vi "Receiver.vi"() -> ()   [LabVIEW 2019]
uses:
  <vilib>/httpClient/LabVIEWHTTPClient.lvlib
  <vilib>/smtpClient/LabVIEWSMTPClient.lvlib
panel:
  out "Data Received, State on/off":bool
  in  "Stop":bool
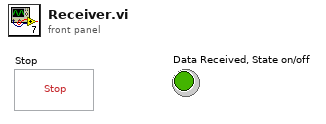
[diagram p1: front panel]
types:
  T1 = typedef "LabVIEWHTTPClient.lvlib/ClientHandle.ctl" = refnum<k1>
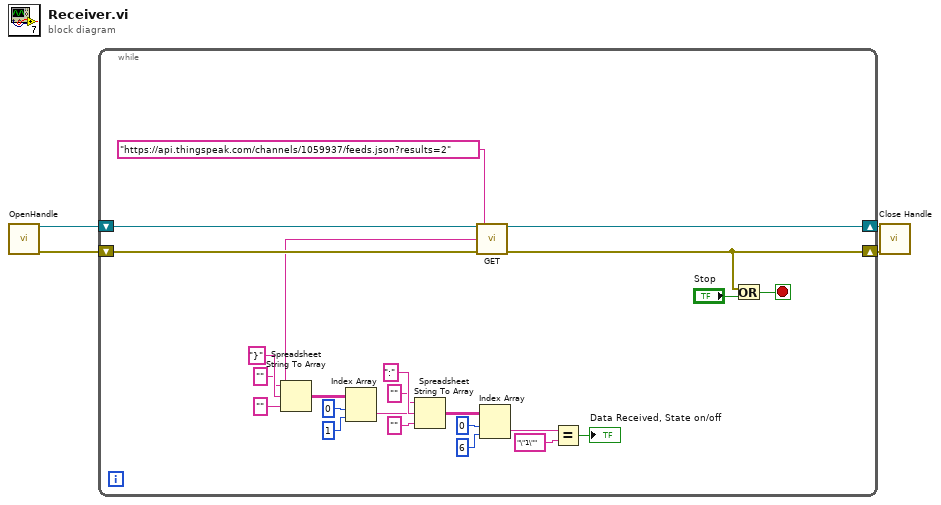
[diagram p0: block diagram]
diagram:
  n1 = call <vilib>:"OpenHandle.vi"() -> ("client handle out"=w4:T1, "error out"=w2:errorcluster)  [unwired: 14 in]
  n2 = while {
    shift-right: [w27] -> w3
    shift-left: w4 -> [w28]
    shift-right: [w5] -> w1
    shift-left: w2 -> [w26]
    stop <- w7 stop-if-true
    n3 = call <vilib>:"GET.vi"("client handle"=w28, "url"="https://api.thingspeak.com/channels/1059937/feeds.json?results=2" ("String"), "error in (no error)"=w26) -> ("client handle out"=w27:T1, "body"=w8:string, "error out"=w5:errorcluster)  [unwired: 9 in, 1 out]
    n4 = Spreadsheet String To Array(delimiter (Tab)="}", format string="", spreadsheet string=w8, array type (2D Dbl)="" ("format string")) -> (array=w18:string[][])
    n5 = Index Array(array=w18, index (row)=0, index (col)=1 ("disabled index (col)")) -> (element=w10:string)
    n6 = Spreadsheet String To Array(delimiter (Tab)=":", format string="", spreadsheet string=w10, array type (2D Dbl)="" ("format string")) -> (array=w13:string[][])
    n7 = Index Array(array=w13, index (row)=0, index (col)=6 ("disabled index (col)")) -> (element=w23:string)
    n8 = Equal?(x=w23, y="\"1\"") -> (x = y?=→"Data Received, State on/off":bool)
    n9 = Or(x=w5, y="Stop") -> (x .or. y?=w7:bool)
  }
  n10 = call <vilib>:"Close Handle.vi"("handle in"=w3, "error in (no error)"=w1) -> ()  [unwired: 12 in, 2 out]
